vi "Record Path.vi"(9 "Record Path":bool) -> ()   [LabVIEW 2020]
uses:
  Framework/Robot Global Data.vi
  <vilib>/Analysis/Matrix/Numeric/Conversions/Matrix To Array - RM.vi
  <vilib>/Utility/file.llb/Write Delimited Spreadsheet (DBL).vi
  <vilib>/Analysis/Matrix/NI_Matrix.lvlib
panel:
  out "Path Counter":dbl
  out "error out":errorcluster
  out "path":path
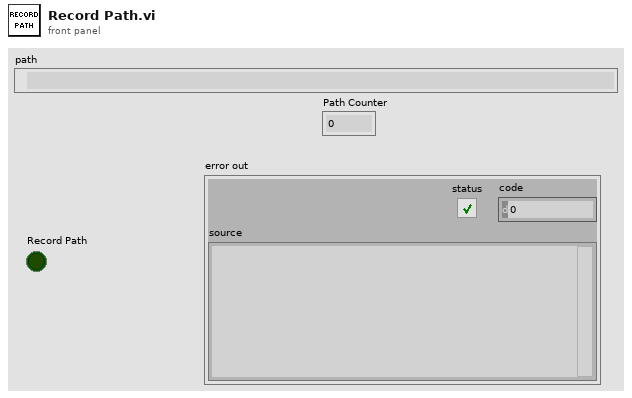
[diagram p1: front panel]
types:
  T1 = typedef "NI_Matrix.lvlib/RealMatrix.ctl" = dbl[][]
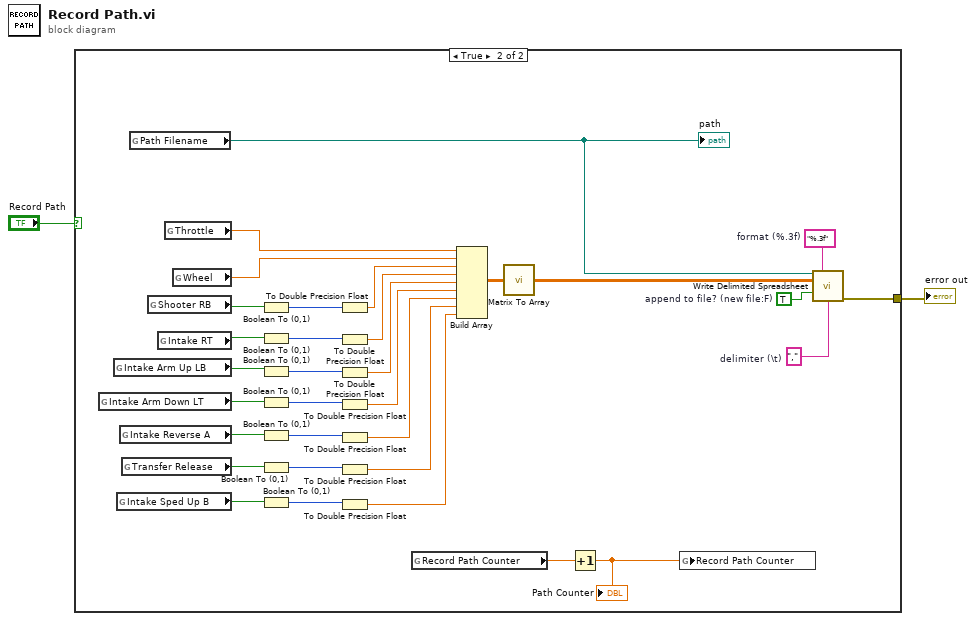
[diagram p0: block diagram]
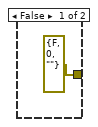
[diagram p2: hidden frame]
diagram:
  n1 = case shown="True" "Record Path" {
    tunnel: [errorcluster {"status"=FALSE, "code"=0, "source"=""} ("error out") w19] -> w1
    frame False {
    }
    frame True {
      w17 = TRUE  # append to file? (new file:F)
      w18 = "%.3f"  # format (%.3f)
      w16 = ","  # delimiter (\t)
      n2 = global read "Robot Global Data.vi" "Intake Arm Down LT"() -> (w20:bool)
      n3 = global read "Robot Global Data.vi" "Intake Arm Up LB"() -> (w21:bool)
      n4 = global read "Robot Global Data.vi" "Intake Sped Up B"() -> (w6:bool)
      n5 = global read "Robot Global Data.vi" "Intake Reverse A"() -> (w12:bool)
      n6 = global read "Robot Global Data.vi" "Transfer Release"() -> (w9:bool)
      n7 = global read "Robot Global Data.vi" "Path Filename"() -> (w15:path)
      "path" <- w15
      n8 = global read "Robot Global Data.vi" "Shooter RB"() -> (w23:bool)
      n9 = global read "Robot Global Data.vi" "Intake RT"() -> (w22:bool)
      n10 = global read "Robot Global Data.vi" "Throttle"() -> (w25:dbl)
      n11 = global read "Robot Global Data.vi" "Wheel"() -> (w24:dbl)
      n12 = Boolean To (0,1)(Boolean=w23) -> (0, 1=w33:i16)
      n13 = Boolean To (0,1)(Boolean=w22) -> (0, 1=w32:i16)
      n14 = Boolean To (0,1)(Boolean=w21) -> (0, 1=w31:i16)
      n15 = Boolean To (0,1)(Boolean=w20) -> (0, 1=w30:i16)
      n16 = Boolean To (0,1)(Boolean=w12) -> (0, 1=w11:i16)
      n17 = Boolean To (0,1)(Boolean=w9) -> (0, 1=w10:i16)
      n18 = Boolean To (0,1)(Boolean=w6) -> (0, 1=w5:i16)
      n19 = To Double Precision Float(number=w33) -> (double precision float=w29:dbl)
      n20 = To Double Precision Float(number=w32) -> (double precision float=w28:dbl)
      n21 = To Double Precision Float(number=w31) -> (double precision float=w27:dbl)
      n22 = To Double Precision Float(number=w30) -> (double precision float=w26:dbl)
      n23 = To Double Precision Float(number=w11) -> (double precision float=w8:dbl)
      n24 = To Double Precision Float(number=w10) -> (double precision float=w7:dbl)
      n25 = To Double Precision Float(number=w5) -> (double precision float=w4:dbl)
      n26 = global read "Robot Global Data.vi" "Record Path Counter"() -> (w14:dbl)
      n27 = Build Array(w25, w24, w29, w28, w27, w26, w8, w7, w4) -> (w35:T1)
      n28 = call-poly <vilib>:"Matrix To Array.vi"("Real Matrix"=w35) -> ("Real 2D Array"=w34:dbl[][])
      n29 = Increment(x=w14) -> (x+1=w13:dbl)
      "Path Counter" <- w13
      n30 = global write "Robot Global Data.vi" "Record Path Counter"(w13) -> ()
      n31 = call-poly <vilib>:"Write Delimited Spreadsheet.vi"("file path (dialog if empty)"=w15, "format (%.3f)"=w18, "2D data"=w34, "append to file? (new file:F)"=w17, "delimiter (\\t)"=w16) -> ("error out"=w19:errorcluster)  [unwired: 9 in, 1 out]
    }
  }
  "error out" <- w1
